vi "subcooled_test.vi"() -> ()   [LabVIEW 2017]
uses:
  <vilib>/Utility/file.llb/Read Delimited Spreadsheet (DBL).vi
panel:
  out "p":dbl
  out "T":dbl
  out "v":dbl
  out "h":dbl
  out "s":dbl
  in  "T Search":dbl
  out "appended path":path
  out "all rows":dbl[][](array[numeric])
  in  "Stop Button":bool
  in  "P Search":dbl
  out "Sat_By_Deg_Arr":dbl[][](array[numeric])
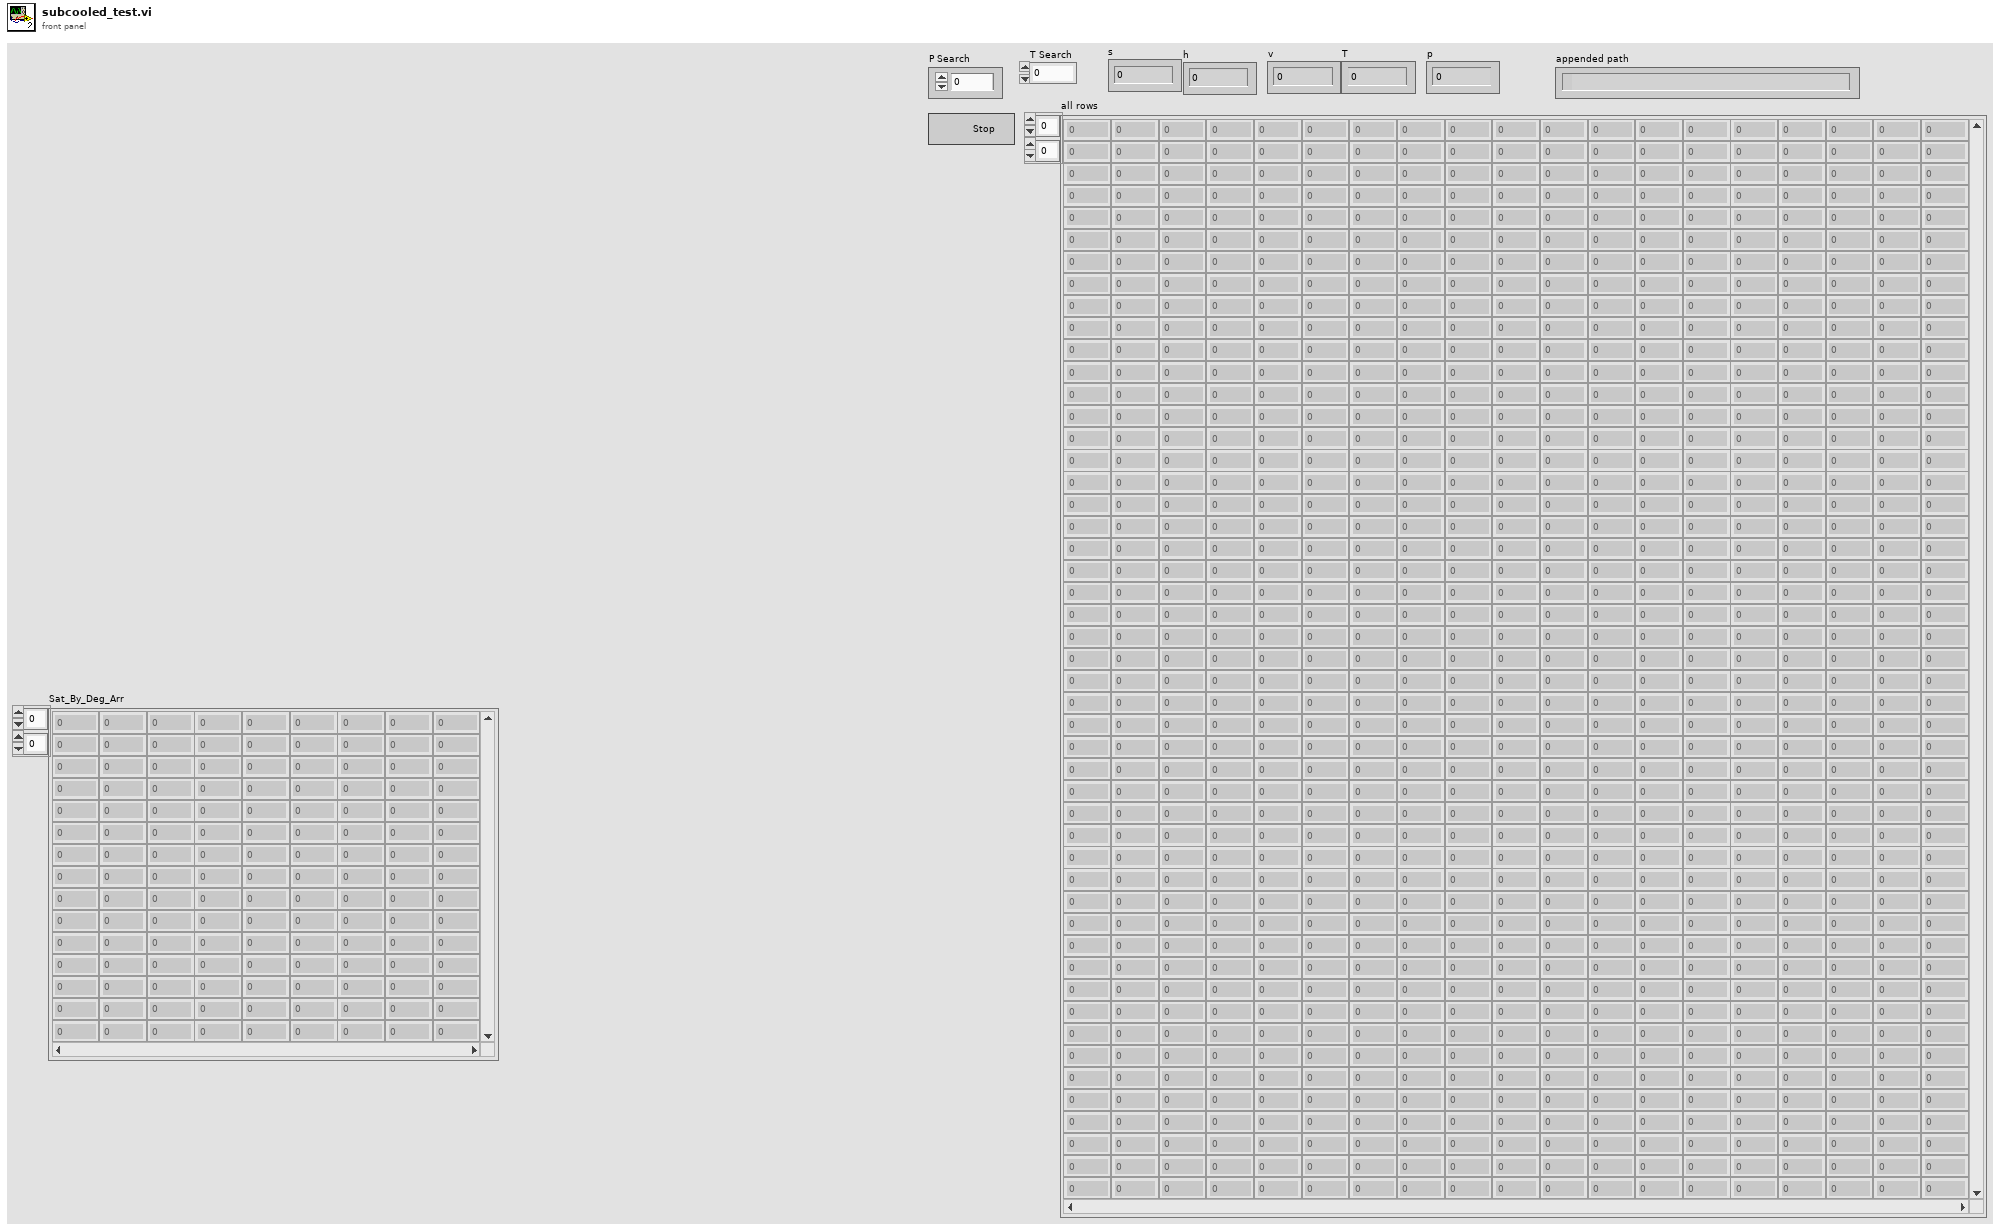
[diagram p1: front panel]
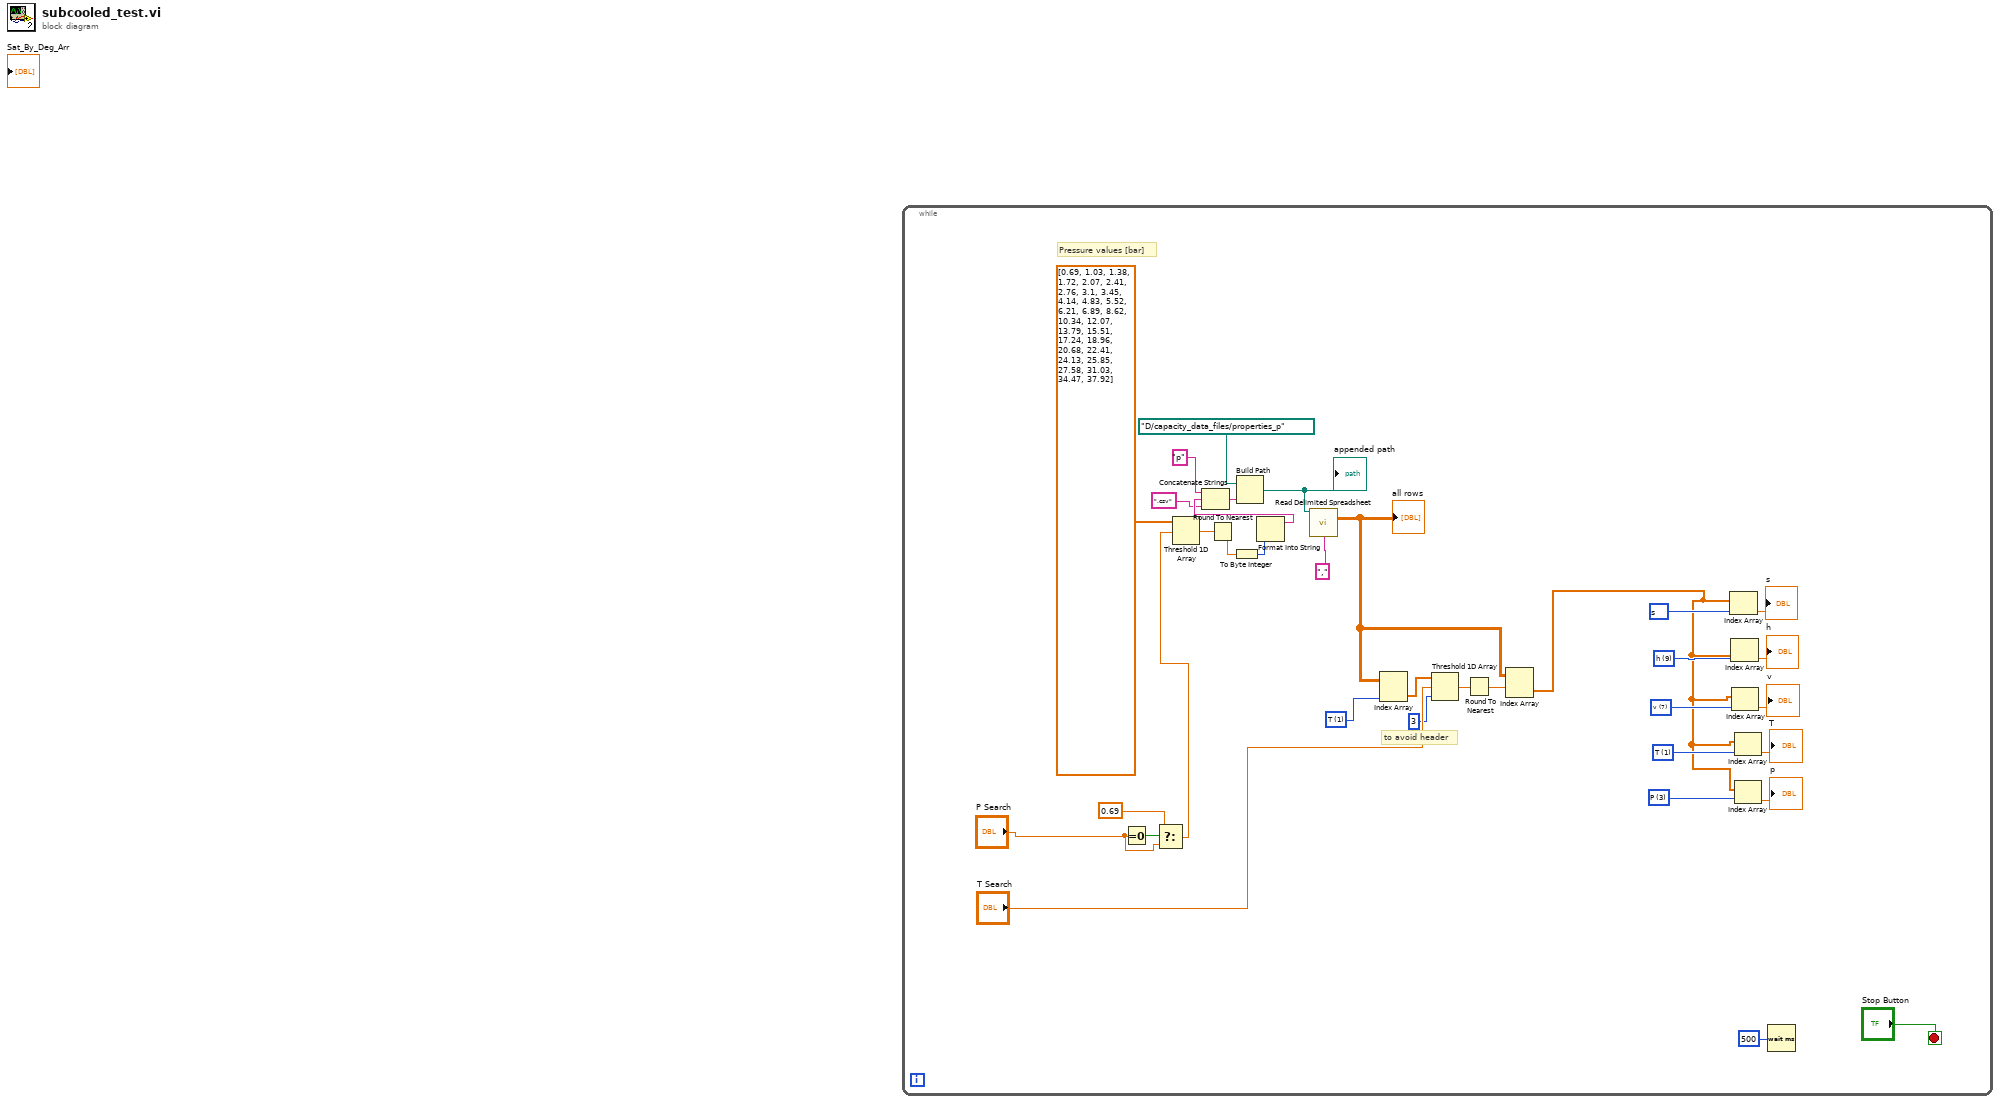
[diagram p0: block diagram]
diagram:
  n1 = while {
    stop <- "Stop Button" stop-if-true
    w8 = u16 1 items=["T"=1, "P"=3, "rho"=5, "v"=7, "h"=9, "s"=11] ("properties columns")
    w18 = u16 1 items=["T"=1, "P"=3, "rho"=5, "v"=7, "h"=9, "s"=11] ("properties columns")
    w10 = u16 3 items=["T"=1, "P"=3, "rho"=5, "v"=7, "h"=9, "s"=11] ("properties columns")
    w9 = u16 9 items=["T"=1, "P"=3, "rho"=5, "v"=7, "h"=9, "s"=11] ("properties columns")
    w11 = u16 7 items=["T"=1, "P"=3, "rho"=5, "v"=7, "h"=9, "s"=11] ("properties columns")
    w12 = u16 11 items=["T"=1, "P"=3, "rho"=5, "v"=7, "h"=9, "s"=11] ("properties columns")
    # "to avoid header"
    # "Pressure values [bar]"
    n2 = Equal To 0?(x="P Search") -> (x = 0?=w34:bool)
    n3 = Select(t=0.69, s=w34, f="P Search") -> (s? t:f=w32:dbl)
    n4 = Threshold 1D Array(2:w32, 3:dbl[] [0.69, 1.03, 1.38, 1.72, 2.07, 2.41, 2.76, 3.1, 3.45, 4.14, 4.83, 5.52, 6.21, 6.89, 8.62, 10.34, 12.07, 13.79, 15.51, 17.24, 18.96, 20.68, 22.41, 24.13, 25.85, 27.58, 31.03, 34.47, 37.92]) -> (0:w31:dbl)  [unwired: 1 in]
    n5 = Round To Nearest(number=w31) -> (nearest integer value=w21:dbl)
    n6 = To Byte Integer(number=w21) -> (8bit integer=w20:i8)
    n7 = Format Into String(w20) -> (resulting string=w27:string)  [unwired: 3 in, 1 out]
    n8 = Concatenate Strings("p" ("string"), w27, ".csv" ("string")) -> (w29:string)
    n9 = Build Path(base path=path "D:/capacity_data_files/properties_p", name or relative path=w29) -> (appended path=w25:path)
    "appended path" <- w25
    n10 = call-poly <vilib>:"Read Delimited Spreadsheet.vi"("file path (dialog if empty)"=w25, "delimiter (\\t)"="," ("delimiter (\\t)")) -> ("all rows"=w14:dbl[][])  [unwired: 8 in, 5 out]
    "all rows" <- w14
    n11 = Index Array(array=w14, index (col)=w18) -> (element=w17:dbl[])  [unwired: 1 in]
    n12 = Threshold 1D Array(1:3 ("start index (0)"), 2:"T Search", 3:w17) -> (0:w15:dbl)
    n13 = Round To Nearest(number=w15) -> (nearest integer value=w13:dbl)
    n14 = Index Array(array=w14, index (row)=w13) -> (element=w7:dbl[])  [unwired: 1 in]
    n15 = Index Array(array=w7, index=w12) -> (element=→"s":dbl)
    n16 = Index Array(array=w7, index=w9) -> (element=→"h":dbl)
    n17 = Index Array(array=w7, index=w11) -> (element=→"v":dbl)
    n18 = Index Array(array=w7, index=w8) -> (element=→"T":dbl)
    n19 = Index Array(array=w7, index=w10) -> (element=→"p":dbl)
    n20 = Wait (ms)(milliseconds to wait=u32 500) -> ()  [unwired: 1 out]
  }
